vi "get_item_by_name.vi"(8 "error in (no error)":errorcluster, 10 "key_name":string, 11 "Table in":refnum<class "InlineTable.lvclass">) -> (0 "error out":errorcluster, 1 "Item":refnum<class "Item.lvclass">, 3 "Table out":refnum<class "InlineTable.lvclass">)   [LabVIEW 2020, in "toml_edit.lvlib" / "InlineTable.lvclass"]
uses:
  InlineTable.lvclass
  Item/Item.lvclass
  InlineTable.lvclass/InlineTable.ctl
  dragon_toml_64.dll
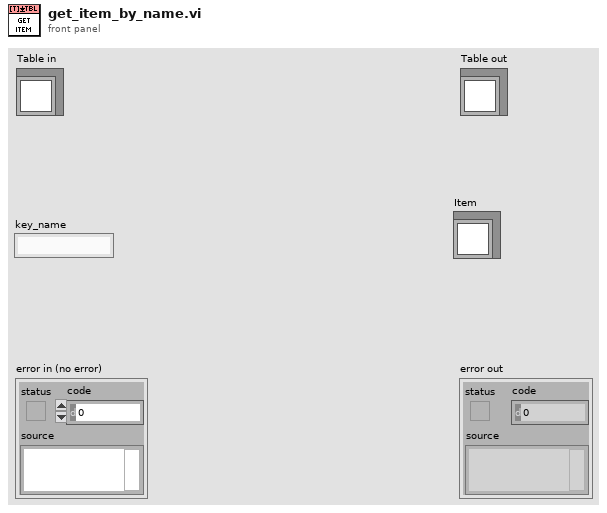
[diagram p1: front panel]
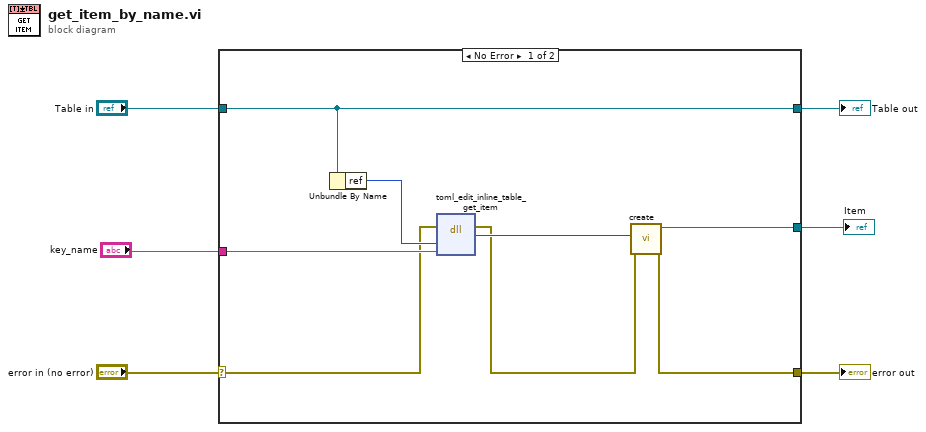
[diagram p0: block diagram]
diagram:
  n1 = case shown="No Error" "error in (no error)" {
    selector: "error in (no error)" -> [w10 w16]
    tunnel: [w7 w16] -> w5
    tunnel: [w13 w15] -> w3
    tunnel: "Table in" -> [w13 w15]
    tunnel: "key_name" -> [w11 _]
    tunnel: [w9 _] -> w1
    frame No Error {
      n2 = Unbundle By Name(w13) -> ("ref"=w12:u64)
      n3 = dll-call lib="C:/Users/JamesMcNally/Documents/toml-edit-labview/lv_src/dragon_toml_*.dll" fn="toml_edit_inline_table_get_item"(error in=w10, "table"=w12, "item_name"=w11) -> (error out=w8:errorcluster, "item"=w14:u64)  [unwired: 4 in, 1 out]
      n4 = call "create.vi"("error in (no error)"=w8, "ref"=w14) -> ("error out"=w7:errorcluster, "Item out"=w9:refnum<class "Item.lvclass">)  [unwired: 7 in, 1 out]
    }
    frame Error {
    }
  }
  "error out" <- w5
  "Table out" <- w3
  "Item" <- w1
